vi "stop_tasks.vi"(8 "error in (no error)":errorcluster, 11 "Experiment in":refnum<class "Experiment.lvclass">) -> (0 "error out":errorcluster, 3 "Experiment out":refnum<class "Experiment.lvclass">)   [LabVIEW 2013, in "Experiment.lvclass"]
uses:
  Experiment.lvclass
  Experiment.lvclass/Experiment.ctl
  Counter/Counter.lvclass
  HSDIO/HSDIO.lvclass
  DAQmx_DO/DAQmx_DO.lvclass
  Analog_output/Analog_Output.lvclass
  Analog_Input/Analog_Input.lvclass
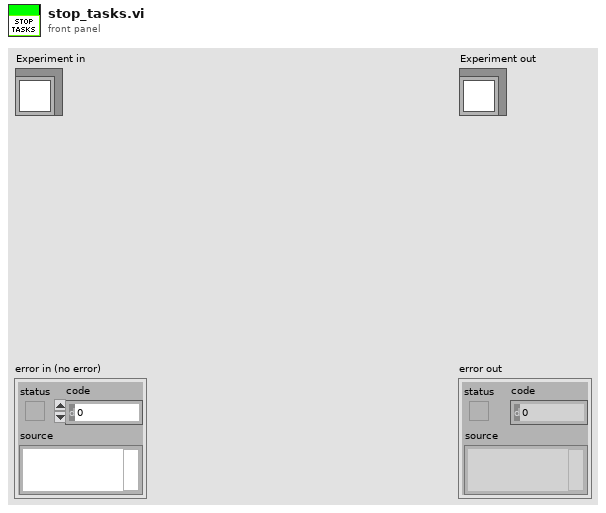
[diagram p1: front panel]
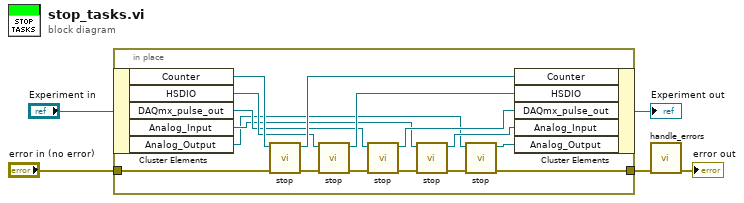
[diagram p0: block diagram]
diagram:
  n1 = in-place {
    in-place-border: "error in (no error)" -> [w15]
    in-place-border: [w13] -> w1
    n2 = in-place-cluster #1("Experiment in") -> ("Counter"=w21:refnum<class "Counter.lvclass">, "HSDIO"=w19:refnum<class "HSDIO.lvclass">, "DAQmx_pulse_out"=w17:refnum<class "DAQmx_DO.lvclass">, "Analog_Input"=w9:refnum<class "Analog_Input.lvclass">, "Analog_Output"=w7:refnum<class "Analog_Output.lvclass">)
    n3 = call-dynamic "stop.vi"("error in (no error)"=w15, "Counter in"=w21) -> ("error out"=w12:errorcluster, "Counter out"=w20:refnum<class "Counter.lvclass">)  [unwired: 8 in]
    n4 = call-dynamic "stop.vi"("error in (no error)"=w12, "HSDIO in"=w19) -> ("error out"=w14:errorcluster, "HSDIO out"=w18:refnum<class "HSDIO.lvclass">)  [unwired: 8 in]
    n5 = call-dynamic "stop.vi"("error in (no error)"=w14, "DAQmx_pulse_out in"=w17) -> ("error out"=w11:errorcluster, "DAQmx_pulse_out out"=w16:refnum<class "DAQmx_DO.lvclass">)  [unwired: 8 in]
    n6 = call "stop.vi"("error in (no error)"=w11, "Analog_Input (in)"=w9) -> ("error out"=w10:errorcluster, "Analog_Input"=w8:refnum<class "Analog_Input.lvclass">)  [unwired: 8 in]
    n7 = call-dynamic "stop.vi"("error in (no error)"=w10, "Analog_Output in"=w7) -> ("error out"=w13:errorcluster, "Analog_Output out"=w6:refnum<class "Analog_Output.lvclass">)  [unwired: 8 in]
    n8 = in-place-cluster #1("Counter"=w20, "HSDIO"=w18, "DAQmx_pulse_out"=w16, "Analog_Input"=w8, "Analog_Output"=w6) -> (→"Experiment out":refnum<class "Experiment.lvclass">)
  }
  n9 = call "handle_errors.vi"("error in (no error)"=w1) -> ("error out"=→"error out":errorcluster)  [unwired: 14 in]
